vi "Get All Installed Files.vi"(8 "Error In":errorcluster, 11 "Configuration":T1) -> (0 "Error Out":errorcluster, 2 "All Installed Files":path[](array[path]), 3 "Configuration":T1)   [LabVIEW 2011, in "LVH-Toolbox.lvlib" / "LVH-Build-Tools.lvlib"]
uses:
  LVH-Build-Tools.lvlib
  Type Defs/Configuration.ctl
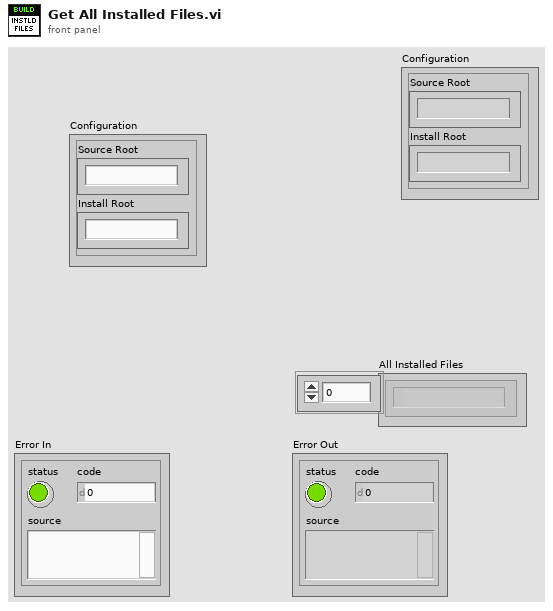
[diagram p1: front panel]
types:
  T1 = typedef "LVH-Toolbox.lvlib/LVH-Build-Tools.lvlib/Configuration.ctl" = cluster{"Source Root":string, "Install Root":string, "Components":string[], "Ignore":string[]}
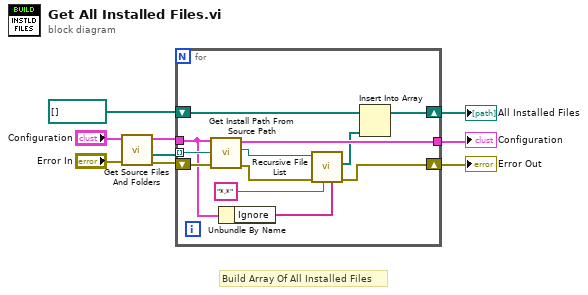
[diagram p0: block diagram]
diagram:
  # "Build Array Of All Installed Files"
  n1 = call "Get Source Files And Folders.vi"("Error In"="Error In", "Configuration"="Configuration") -> ("Error Out"=w6:errorcluster, "All Source Folders"=w5:path[], "Configuration"=w9:T1)  [unwired: 6 in, 1 out]
  n2 = for {
    tunnel: w5 -> [w20] mode=indexing
    tunnel: w9 -> [w15]
    shift-right: [w13] -> w2
    shift-left: w6 -> [w21]
    tunnel: [w19] -> w1
    shift-right: [w11] -> w4
    shift-left: path[] [] ("Array in") -> [w12]
    n3 = call "Get Install Path From Source Path.vi"("Error In"=w21, "Source File Path"=w20, "Configuration"=w15) -> ("Error Out"=w17:errorcluster, "Install File Path"=w18:path, "Configuration"=w19:T1)  [unwired: 5 in, 1 out]
    n4 = Unbundle By Name(w15) -> ("Ignore"=w14:string[])
    n5 = call <vilib>:"Recursive File List.vi"("Folders to Exclude"=w14, "pattern"="*.*", "error in (no error)"=w17, "Folder Path"=w18) -> ("error out"=w13:errorcluster, "All Files in Dir"=w10:path[])  [unwired: 3 in, 3 out]
    n6 = Insert Into Array(array=w12, new element=w10) -> (w11:path[])  [unwired: 1 in]
  }
  "All Installed Files" <- w4
  "Error Out" <- w2
  "Configuration" <- w1
